vi "Convolute Signals.vi"(0 "reference in":refnum<class "SigMath.lvclass">, 5 "error in (no error)":errorcluster, 6 "Operation Option":enum16{"Convolute", "DE-Convolute"}(ring), 7 "Sub Signals A":i32[](listbox) caption="Set A", 9 "Sub Signals B":i32[](listbox) caption="Set B") -> (14 "reference out":refnum<class "SigMath.lvclass">, 19 "error out":errorcluster)   [LabVIEW 2022 SP3, in "SigMath.lvclass"]
uses:
  SigMath.lvclass
  API/GSwFormDSP_class/functions/Attribute List.ctl
  API/GSwFormDSP_class/functions/Attribute Options.ctl
  <vilib>/Analysis/2dsp.llb/1D Convolution (DBL).vi
  API/GSwFormDSP_class/GSwFormDSP.lvclass
  <vilib>/Analysis/NI_AALPro.lvlib
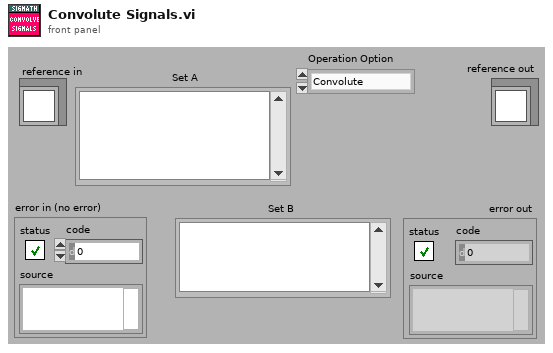
[diagram p1: front panel]
types:
  T1 = typedef "GSwFormDSP.lvclass/Attribute Options.ctl" = enum16{"Append to Attribute using \"( )\"", "Replace Attribute Value"}
  T2 = typedef "GSwFormDSP.lvclass/Attribute List.ctl" = string
  T3 = typedef "SigMath.lvclass/ObjectAttributes.ctl" = cluster{"SigMath Data":T4, "User CTRL Refs":T5}
  T4 = typedef "SigMath.lvclass/SigMath Data.ctl" = cluster{"New Time Data Obj?":bool, "GSwFormDSP":refnum<class "GSwFormDSP.lvclass">}
  T5 = typedef "SigMath.lvclass/SigMath User CTRL Refs.ctl" = cluster{"wForms":refnum<vi>, "Results wForms":refnum<vi>}
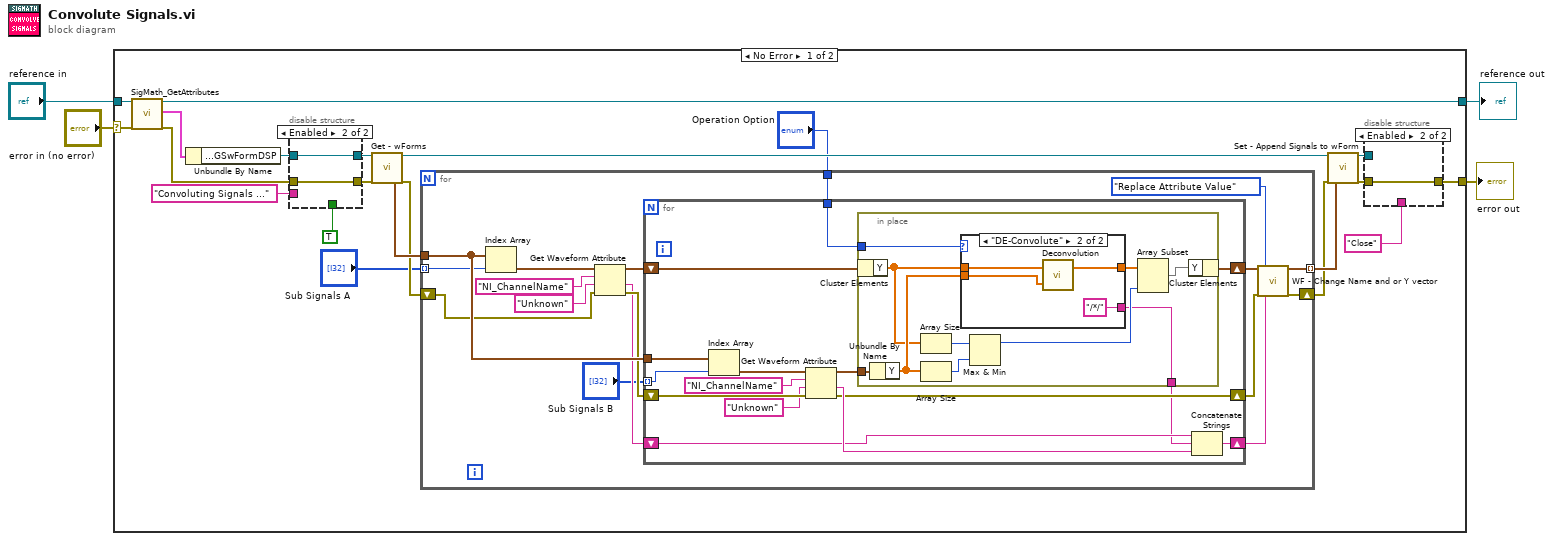
[diagram p0: block diagram]
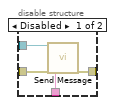
[diagram p2: hidden frame]
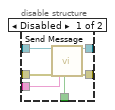
[diagram p3: hidden frame]
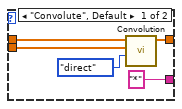
[diagram p4: hidden frame]
diagram:
  n1 = case shown="No Error" "error in (no error)" {
    selector: "error in (no error)" -> [w25 w91]
    tunnel: [w7 w91] -> w3
    tunnel: [w24 w90] -> w1
    tunnel: "reference in" -> [w23 w90]
    frame No Error {
      n2 = call "SigMath_GetAttributes.vi"("reference in"=w23, "error in (no error)"=w25) -> ("reference out"=w24:refnum<class "SigMath.lvclass">, "attributes"=w22:T3, "error out"=w12:errorcluster)  [unwired: 14 in, 1 out]
      n3 = Unbundle By Name(w22) -> ("SigMath Data.GSwFormDSP"=w15:refnum<class "GSwFormDSP.lvclass">)
      n4 = disable-structure shown="Enabled" {
        disable-tunnel: w15 -> [w36 w38]
        disable-tunnel: [w35 w38] -> w14
        disable-tunnel: [w34 w37] -> w13
        disable-tunnel: w12 -> [w33 w37]
        disable-tunnel: TRUE ("Make Cursor Busy?") -> [w32 _]
        disable-tunnel: "Convoluting Signals ..." ("Message (\"\" closes the window)") -> [w31 _]
        frame Disabled {
          n5 = call-dynamic "Send Message.vi"("reference in"=w36, "error in (no error)"=w33, "Message (\"\" closes the window)"=w31, "Make Cursor Busy?"=w32) -> ("reference out"=w35:refnum<class "GSwFormDSP.lvclass">, "error out"=w34:errorcluster)  [unwired: 14 in]
        }
        frame Enabled {
        }
      }
      n6 = call-dynamic "Get - wForms.vi"("reference in"=w14, "error in (no error)"=w13) -> ("wForms"=w21:waveform(dbl)[], "reference out"=w20:refnum<class "GSwFormDSP.lvclass">, "error out"=w18:errorcluster)  [unwired: 14 in, 1 out]
      n7 = for {
        tunnel: w21 -> [w55]
        tunnel: [w42] -> w19 mode=indexing
        shift-right: [w43] -> w17
        shift-left: w18 -> [w50]
        tunnel: "Sub Signals A" -> [w41] mode=indexing
        tunnel: "Operation Option" -> [w39]
        n8 = Index Array(array=w55, index=w41) -> (element=w53:waveform(dbl))
        n9 = Get Waveform Attribute(4:w50, 5:"Unknown", 6:T2 "NI_ChannelName" ("Attribute List"), 7:w53) -> (0:w49:errorcluster, 1:w48:string, 3:w52:waveform(dbl))  [unwired: 1 out]
        n10 = for {
          shift-right: [w58] -> w47
          shift-left: w52 -> [w60]
          tunnel: w55 -> [w70]
          shift-right: [w59] -> w45
          shift-left: w49 -> [w68]
          shift-right: [w63] -> w44
          shift-left: w48 -> [w64]
          tunnel: "Sub Signals B" -> [w61] mode=indexing
          tunnel: w39 -> [w57]
          n11 = Index Array(array=w70, index=w61) -> (element=w69:waveform(dbl))
          n12 = Get Waveform Attribute(4:w68, 5:"Unknown", 6:T2 "NI_ChannelName" ("Attribute List"), 7:w69) -> (0:w59:errorcluster, 1:w65:string, 3:w62:waveform(dbl))  [unwired: 1 out]
          n13 = in-place {
            in-place-border: w62 -> [w80]
            in-place-border: w57 -> [w72]
            in-place-border: [w71] -> w56
            n14 = in-place-cluster #1(w60) -> ("Y"=w78:dbl[])
            n15 = Unbundle By Name(w80) -> ("Y"=w79:dbl[])
            n16 = Array Size(array=w78) -> (size(s)=w77:i32)
            n17 = Array Size(array=w79) -> (size(s)=w76:i32)
            n18 = case shown="\"DE-Convolute\"" w72 {
              tunnel: w79 -> [w84 w87]
              tunnel: w78 -> [w83 w88]
              tunnel: [w82 w89] -> w75
              tunnel: ["*" ("string") "/*/" ("string")] -> w71
              frame "Convolute", Default {
                n19 = call-poly <vilib>:"Convolution.vi"("algorithm"=enum32{"direct", "frequency domain"}."direct", "Y"=w84, "X"=w83) -> ("X * Y"=w82:dbl[])  [unwired: 7 in, 1 out]
              }
              frame "DE-Convolute" {
                n20 = call <vilib>:"Deconvolution.vi"("Y"=w87, "X * Y"=w88) -> ("X"=w89:dbl[])  [unwired: 1 out]
              }
            }
            n21 = Max & Min(x=w77, y=w76) -> (max(x,y)=w74:i32)  [unwired: 1 out]
            n22 = Array Subset(array=w75, length=w74) -> (w73:dbl[])  [unwired: 1 in]
            n23 = in-place-cluster #1("Y"=w73) -> (w58:waveform(dbl))
          }
          n24 = Concatenate Strings(w64, w56, w65) -> (w63:string)
        }
        n25 = call "WF - Change Name and or Y vector.vi"("wForm IN"=w47, "error in (no error)"=w45, "Attribute Option"=Attribute_Options."Replace Attribute Value", "SigName Update"=w44) -> ("wForm OUT"=w42:waveform(dbl), "error out"=w43:errorcluster)  [unwired: 14 in]
      }
      n26 = call "Set - Append Signals to wForm.vi"("reference in"=w20, "error in (no error)"=w17, "New Signals"=w19) -> ("reference out"=w9:refnum<class "GSwFormDSP.lvclass">, "error out"=w8:errorcluster)  [unwired: 15 in]
      n27 = disable-structure shown="Enabled" {
        disable-tunnel: w9 -> [w29 _]
        disable-tunnel: w8 -> [w28 w30]
        disable-tunnel: [w27 w30] -> w7
        disable-tunnel: "Close" ("Message (\"\" closes the window)") -> [w26 _]
        frame Disabled {
          n28 = call-dynamic "Send Message.vi"("reference in"=w29, "error in (no error)"=w28, "Message (\"\" closes the window)"=w26) -> ("error out"=w27:errorcluster)  [unwired: 15 in, 1 out]
        }
        frame Enabled {
        }
      }
    }
    frame Error {
    }
  }
  "error out" <- w3
  "reference out" <- w1
